vi "Create Status Variables.vi"(8 "error in (no error)":errorcluster, 11 "System Configuration":T1) -> (0 "error out":errorcluster, 3 "dup System Configuration":T1)   [LabVIEW 2024]
doc: "Creates shared variables that indicate the server status."
uses:
  Controls/Server/System Configuration.ctl
  Controls/Server/Subsystem Configuration.ctl
  <vilib>/lvdsc/NI_DSC.lvlib
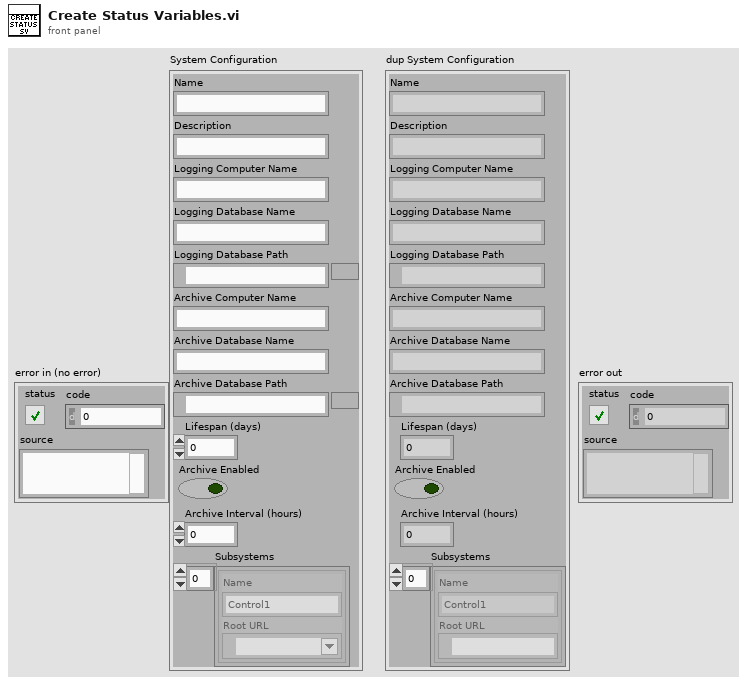
[diagram p1: front panel]
types:
  T1 = typedef "System Configuration.ctl" = cluster{"Name":string, "Description":string, "Logging Computer Name":string, "Logging Database Name":string, "Logging Database Path":path, "Archive Computer Name":string, "Archive Database Name":string, "Archive Database Path":path, "Lifespan (days)":u32, "Archive Enabled":bool, "Archive Interval (hours)":u32, "Subsystems":T2[]}
  T2 = typedef "Subsystem Configuration.ctl" = cluster{"Name":string, "Root URL":refnum<k21>}
  T3 = enum32{"u32BitField", "bool", "double", "string", "int8", "uint8", "int16", "uint16", "int32", "uint32", "int64", "uint64", "single", "double waveform", "int16 waveform", "array of boolean", "array of int8", "array of uint8", "array of int16", "array of uint16", "array of int32", "array of uint32", "array of int64", "array of uint64", "array of single", "array of double", "array of double waveform", "array of int16 waveform", "array of string", "variant", "timestamp", "fixed point", "custom"}
  T4 = cluster{"enable? (F)":bool, "data type (deprecated)":enum32{"U32 Bit Field", "Boolean", "Double", "String"}, "initial value":variant}
  T5 = cluster{"format string":string, "data type":enum32{"u32BitField", "bool", "double", "string", "int8", "uint8", "int16", "uint16", "int32", "uint32", "int64", "uint64", "single", "double waveform", "int16 waveform", "array of boolean", "array of int8", "array of uint8", "array of int16", "array of uint16", "array of int32", "array of uint32", "array of int64", "array of uint64", "array of single", "array of double", "array of double waveform", "array of int16 waveform", "array of string", "variant", "timestamp", "fixed point", "custom"}}
  T6 = cluster{"format string":string, "data type":enum32{"u32BitField", "bool", "double", "string", "int8", "uint8", "int16", "uint16", "int32", "uint32", "int64", "uint64", "single", "double waveform", "int16 waveform", "array of boolean", "array of int8", "array of uint8", "array of int16", "array of uint16", "array of int32", "array of uint32", "array of int64", "array of uint64", "array of single", "array of double", "array of double waveform", "array of int16 waveform", "array of string", "variant", "timestamp", "fixed point", "custom"}}[]
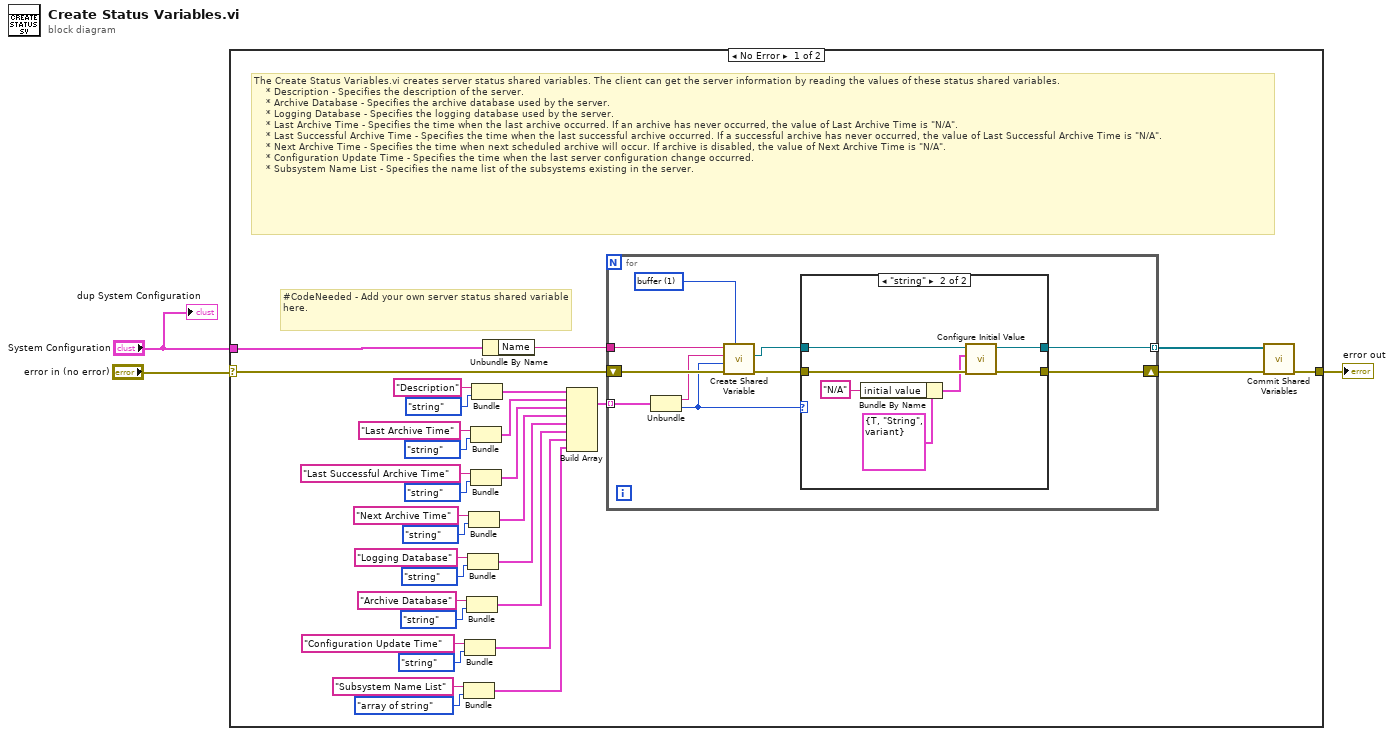
[diagram p0: block diagram]
diagram:
  n1 = case shown="No Error" "error in (no error)" {
    selector: "error in (no error)" -> [w31 w54]
    tunnel: [w34 w54] -> w3
    tunnel: "System Configuration" -> [w29 _]
    frame No Error {
      # "#CodeNeeded - Add your own server status shared variable here."
      # "The Create Status Variables.vi creates server status shared variables. The client can get the server information by reading the values of these status shared variables.\n    * Description - Specifies the description of the server.\n    * Archive Database - Specifies the archive database used by the server. \n    * Logging Database - Specifies the logging database used by the server.\n    * Last Archive Time - Specifies the time when the last archive occurred. If an archive has never occurred, the value of Last Archive Time is \"N/A\".\n    * Last Successful Archive Time - Specifies the time when the last successful archive occurred. If a successful archive has never occurred, the value of Last Successful Archive Time is \"N/A\".\n    * Next Archive Time - Specifies the time when next scheduled archive will occur. If archive is disabled, the value of Next Archive Time is \"N/A\".\n    * Configuration Update Time - Specifies the time when the last server configuration change occurred.\n    * Subsystem Name List - Specifies the name list of the subsystems existing in the server."
      n2 = Bundle("format string"="Subsystem Name List", "data type"=T3."array of string") -> (w4:T5)  [unwired: 1 in]
      n3 = Bundle("format string"="Configuration Update Time", "data type"=T3."string") -> (w5:T5)  [unwired: 1 in]
      n4 = Bundle("format string"="Archive Database", "data type"=T3."string") -> (w10:T5)  [unwired: 1 in]
      n5 = Bundle("format string"="Logging Database", "data type"=T3."string") -> (w13:T5)  [unwired: 1 in]
      n6 = Bundle("format string"="Next Archive Time", "data type"=T3."string") -> (w16:T5)  [unwired: 1 in]
      n7 = Bundle("format string"="Last Archive Time", "data type"=T3."string") -> (w22:T5)  [unwired: 1 in]
      n8 = Bundle("format string"="Last Successful Archive Time", "data type"=T3."string") -> (w19:T5)  [unwired: 1 in]
      n9 = Bundle("format string"="Description", "data type"=T3."string") -> (w25:T5)  [unwired: 1 in]
      n10 = Unbundle By Name(w29) -> ("Name"=w28:string)
      n11 = Build Array(w25, w22, w19, w16, w13, w10, w5, w4) -> (w30:T6)
      n12 = for {
        tunnel: w30 -> [w37] mode=indexing
        tunnel: [w41] -> w33 mode=indexing
        shift-right: [w40] -> w32
        shift-left: w31 -> [w42]
        tunnel: w28 -> [w38]
        w39 = u16 1 items=["commit", "buffer"] ("set mode")
        n13 = Unbundle(w37) -> ("format string"=w36:string, "data type"=w35:T3)
        n14 = call <vilib>:"Create Shared Variable.vi"("set mode"=w39, "error in (no error)"=w42, "data type"=w35, "shared variable name"=w36, "process name"=w38) -> ("error out"=w43:errorcluster, "shared variable"=w44:refnum<k21>)  [unwired: 4 in, 1 out]
        n15 = case shown="\"string\"" w35 {
          tunnel: w44 -> [w46 w53]
          tunnel: w43 -> [w45 w52]
          tunnel: [w46 w51] -> w41
          tunnel: [w45 w50] -> w40
          frame Default {
          }
          frame "string" {
            n16 = Bundle By Name(cluster=T4 {"enable? (F)"=TRUE, "data type (deprecated)"=enum."String", "initial value"=variant} ("initial value settings"), "initial value"="N/A" ("format string")) -> (w47:T4)
            n17 = call <vilib>:"Configure Initial Value.vi"("error in (no error)"=w52, "initial value settings"=w47, "variable reference in"=w53) -> ("error out"=w50:errorcluster, "variable reference out"=w51:refnum<k21>)  [unwired: 7 in]
          }
        }
      }
      n18 = call <vilib>:"Commit Shared Variables.vi"("error in (no error)"=w32, "shared variables"=w33) -> ("error out"=w34:errorcluster)  [unwired: 9 out]
    }
    frame Error {
    }
  }
  "error out" <- w3
  "dup System Configuration" <- "System Configuration"
